vi "Update Results.vi"(0 "measurement service v2 in":refnum<class "Measurement Service V2.lvclass">, 5 "measurement results":variant, 7 "measurement plugin service in":refnum<class "Measurement Plugin Service.lvclass">, 9 "gRPC ID in":T1, 11 "error in":errorcluster) -> (4 "measurement service v2 out":refnum<class "Measurement Service V2.lvclass">, 8 "measurement plugin service out":refnum<class "Measurement Plugin Service.lvclass">, 15 "error out":errorcluster)   [LabVIEW 2020, in "MeasurementLink Measurement Server.lvlib" / "Measurement Service V2.lvclass"]
uses:
  Measurement Service V2.lvclass
  <vilib>/gRPC/LabVIEW gRPC Library/Shared/grpcId.ctl
  Measurement Plugin Service/Measurement Plugin Service.lvclass
  Generated/Measurement Plugin Measurement Service Base V2/RPC Messages/ni_measurementlink_measurement_v2_MeasureResponse.ctl
  Generated/Measurement Plugin Measurement Service Base V2/RPC Messages/google_protobuf_Any.ctl
  Generated/Measurement Plugin Measurement Service Base V2/RPC Service/MeasurementService/MeasurementServiceBaseV2.lvclass
  Generated/Measurement Plugin Measurement Service Base V2/Measurement Plugin Measurement Service Base V2.lvlib
  <vilib>/gRPC/LabVIEW gRPC Library/grpc-lvsupport-release.lvlib
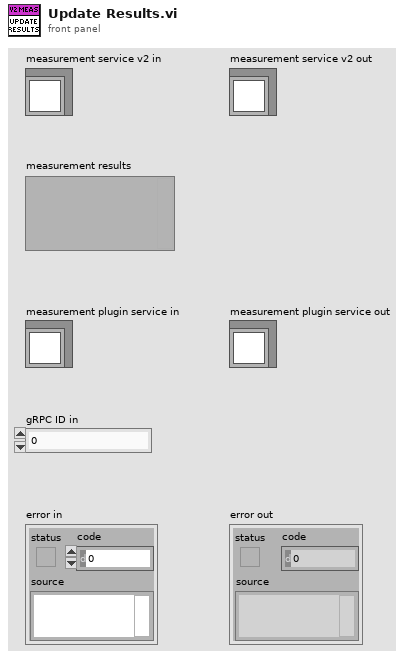
[diagram p1: front panel]
types:
  T1 = typedef "grpc-lvsupport-release.lvlib/grpcId.ctl" = u64
  T2 = typedef "Measurement Plugin Measurement Service Base V2.lvlib/ni_measurementlink_measurement_v2_MeasureResponse.ctl" = cluster{"outputs":T3}
  T3 = typedef "Measurement Plugin Measurement Service Base V2.lvlib/google_protobuf_Any.ctl" = cluster{"type_url":string, "value":u8[]}
  T4 = typedef "grpc-lvsupport-release.lvlib/Any.ctl" = cluster{"Type Url":string, "Bytes":u8[]}
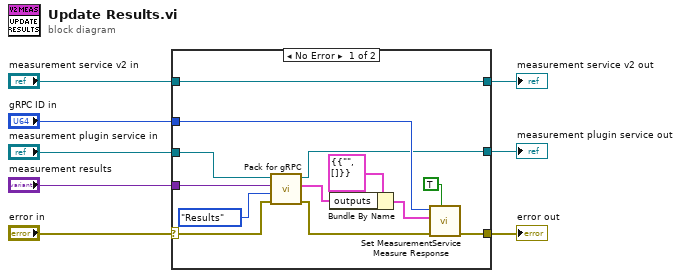
[diagram p0: block diagram]
diagram:
  n1 = case shown="No Error" "error in" {
    selector: "error in" -> [w14 w24]
    tunnel: [w21 w24] -> w7
    tunnel: [w18 w23] -> w5
    tunnel: "measurement service v2 in" -> [w18 w23]
    tunnel: "measurement results" -> [w16 _]
    tunnel: "gRPC ID in" -> [w19 _]
    tunnel: "measurement plugin service in" -> [w17 w22]
    tunnel: [w12 w22] -> w1
    frame No Error {
      n2 = call-dynamic "Pack for gRPC.vi"("error in"=w14, "configuration / results"=enum16{"Configuration", "Results"}."Results" ("Configuration / Resuls (Config)"), "data value"=w16, "measurement plugin service in"=w17) -> ("error out"=w13:errorcluster, "any"=w10:T4, "measurement plugin service out"=w12:refnum<class "Measurement Plugin Service.lvclass">)  [unwired: 5 in]
      n3 = Bundle By Name(cluster=T2 {"outputs"={"type_url"="", "value"=[]}} ("Message Data"), "outputs"=w10) -> (w9:T2)
      n4 = call "Set MeasurementService Measure Response.vi"("Streaming? (F)"=TRUE, "error in (no error)"=w13, "Message Data"=w9, "gRPCid in"=w19) -> ("error out"=w21:errorcluster)  [unwired: 7 in]
    }
    frame Error {
    }
  }
  "error out" <- w7
  "measurement service v2 out" <- w5
  "measurement plugin service out" <- w1
